vi "ZFINAL.vi"() -> ()   [LabVIEW 2014]
panel:
  in  "OK Button 4":bool caption="OK Button 3"
  out "USB Missing 6":bool
  out "USB Missing 5":bool
  in  "OK Button 3":bool
  in  "OK Button 2":bool
  in  "stop":bool
  in  "XY and Servo":bool
  out "USB Missing 4":bool
  out "USB Detected 4":bool
  out "USB Missing 3":bool
  out "USB Detected 3":bool
  out "USB Missing 2":bool
  out "USB Detected 2":bool
  out "USB Missing":bool
  out "USB Detected":bool
  out "Image":T1(plugin-control)
  # "Free-kick Kicker"
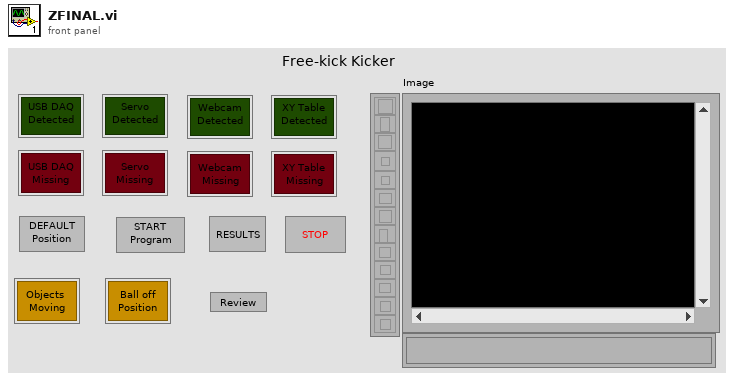
[diagram p1: front panel]
types:
  T1 = typedef "IMAQ Image.ctl" = refnum<image>
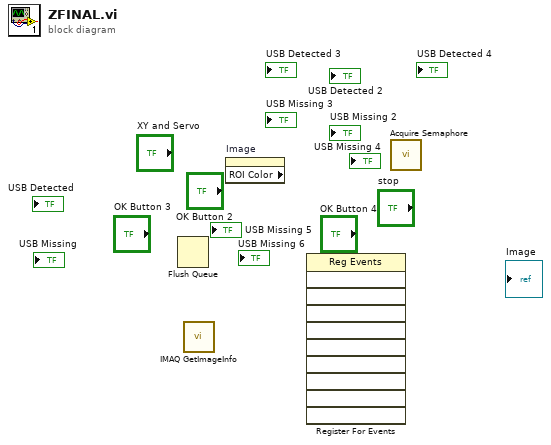
[diagram p0: block diagram]
diagram:
  n1 = Flush Queue() -> ()  [unwired: 2 in, 3 out]
  n2 = call "IMAQ GetImageInfo"() -> ()  [unwired: 4 in, 8 out]
  n3 = property on="Image" class="ImageControl" props=["ROI Color"]() -> ()  [unwired: 2 in, 3 out]
  n4 = register-events() -> ()  [unwired: 11 in, 2 out]
  n5 = call <vilib>:"Acquire Semaphore.vi"() -> ()  [unwired: 5 in, 3 out]
